vi "Calculate Theta Error.vi"(8 "yError":dbl, 9 "xError":dbl, 10 "heading":dbl) -> (2 "thetaError":dbl)   [LabVIEW 2017]
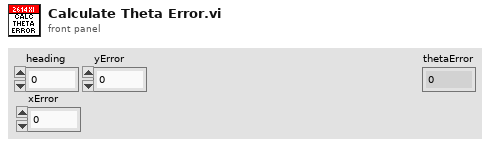
[diagram p1: front panel]
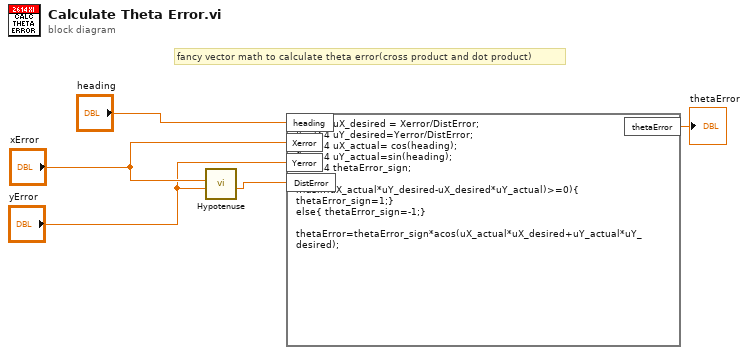
[diagram p0: block diagram]
diagram:
  # "fancy vector math to calculate theta error(cross product and dot product)"
  n1 = call "Hypotenuse.vi"("b"="yError", "a"="xError") -> ("c"=w2:dbl)  [unwired: 9 in]
  n2 = formula code="float64 uX_desired = Xerror/DistError;\nfloat64 uY_desired=Yerror/DistError;\nfloat64 uX_actual= cos(heading);\nfloat64 uY_actual=sin(heading);\nfloat64 thetaError_sign;\n\nif(asin(uX_actual*uY_desired-uX_desired*uY_actual)>=0){\nthetaError_sign=1;} \nelse{ thetaError_sign=-1;}\n\nthetaError=thetaError_sign*acos(uX_actual*uX_desired+uY_actual*uY_desired);"("heading"="heading", "Xerror"="xError", "Yerror"="yError", "DistError"=w2) -> ("thetaError"=→"thetaError":dbl)
